vi "Calculate angle of intersection(Circle).vi"(8 "error in (no error)":errorcluster, 9 "Circle":T1, 10 "Pixel density":dbl format="%#_13g", 11 "Input point":cluster{"X":sgl, "Y":sgl}) -> (0 "error out":errorcluster, 1 "Sleeping line start point":cluster{"X":sgl, "Y":sgl}, 2 "slanting line start poing":cluster{"X":sgl, "Y":sgl}, 3 "Angle":sgl)   [LabVIEW 2019]
uses:
  <vilib>/vision/NI_Vision_Development_Module.lvlib
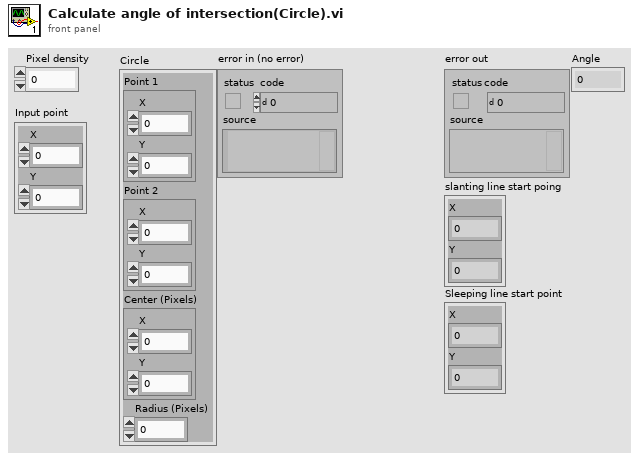
[diagram p1: front panel]
types:
  T1 = cluster{"Point 1":cluster{"X":sgl, "Y":sgl}, "Point 2":cluster{"X":sgl, "Y":sgl}, "Center (Pixels)":cluster{"X":sgl, "Y":sgl}, "Radius (Pixels)":dbl}
  T2 = cluster{"Origin":cluster{"X":sgl, "Y":sgl}, "Angle (deg)":sgl, "Axis Reference":u32}
  T3 = typedef "ROI Descriptor" = cluster{"Global Rectangle":i32[], "Contours":cluster{"ID":enum32{"External", "Internal"}, "Type":u32, "Coordinates":i32[]}[]}
  T4 = typedef "IMAQ Point" = cluster{"X":sgl, "Y":sgl}
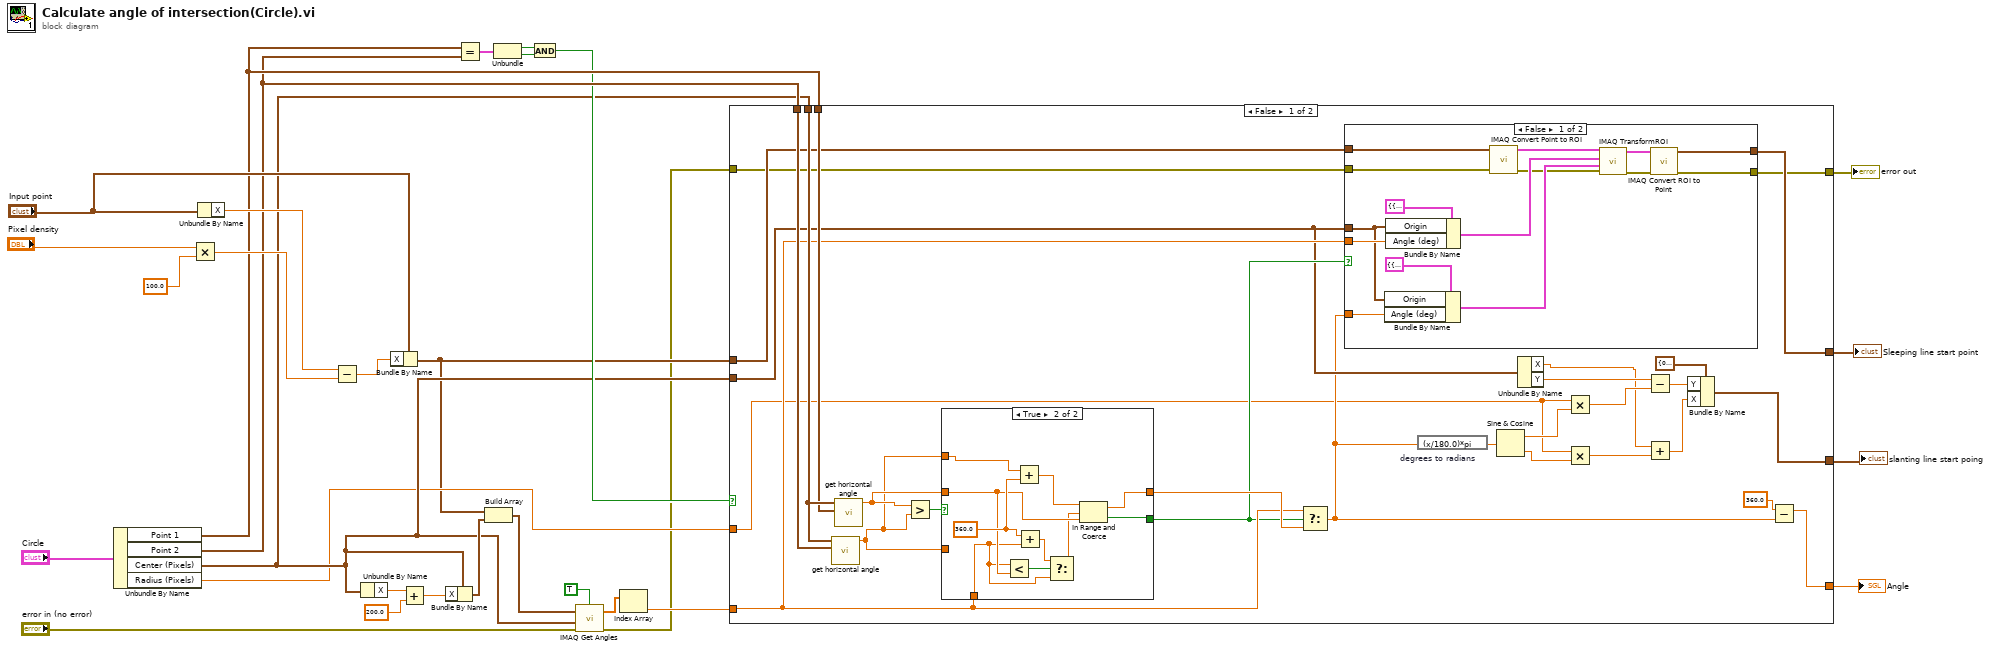
[diagram p0: block diagram]
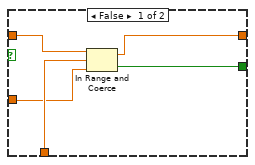
[diagram p3: hidden frame]
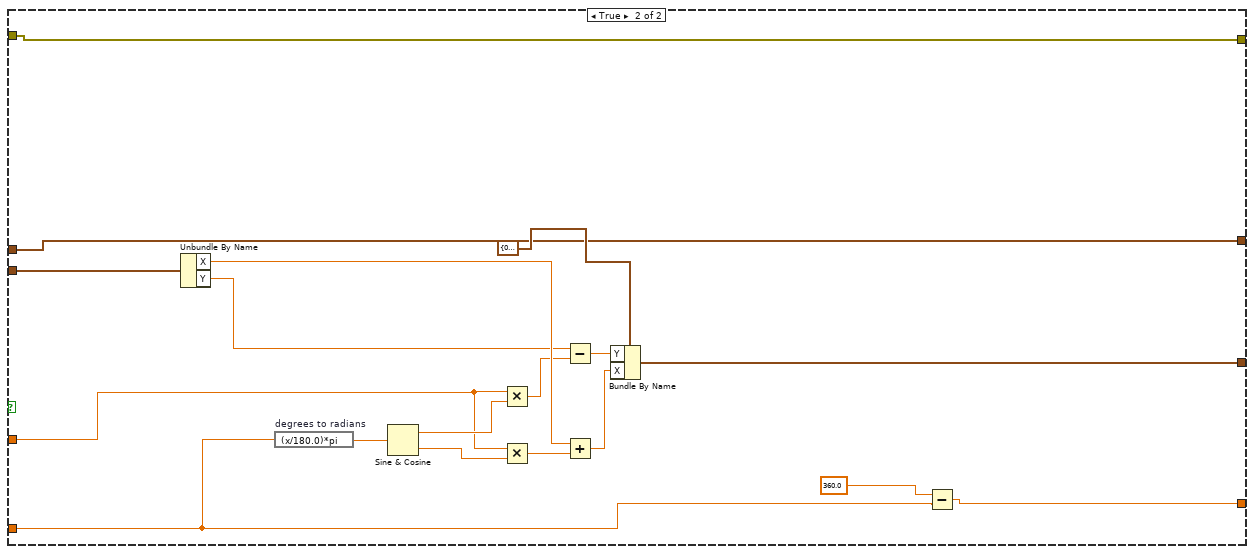
[diagram p4: hidden frame]
diagram:
  n1 = Unbundle By Name("Circle") -> ("Point 1"=w15:cluster{"X":sgl, "Y":sgl}, "Point 2"=w14:cluster{"X":sgl, "Y":sgl}, "Center (Pixels)"=w8:cluster{"X":sgl, "Y":sgl}, "Radius (Pixels)"=w7:dbl)
  n2 = Multiply(x="Pixel density", y=100.0) -> (x*y=w27:dbl)
  n3 = Unbundle By Name("Input point") -> ("X"=w28:sgl)
  n4 = Subtract(x=w28, y=w27) -> (x-y=w25:dbl)
  n5 = Unbundle By Name(w8) -> ("X"=w23:sgl)
  n6 = Bundle By Name(cluster="Input point", "X"=w25) -> (w5:cluster{"X":sgl, "Y":sgl})
  n7 = Add(x=w23, y=sgl 200.0) -> (x+y=w21:sgl)
  n8 = Bundle By Name(cluster=w8, "X"=w21) -> (w19:cluster{"X":sgl, "Y":sgl})
  n9 = Equal?(x=w15, y=w14) -> (x = y?=w13:cluster{"X":bool, "Y":bool})
  n10 = Build Array(w5, w19) -> (w20:cluster{"X":sgl, "Y":sgl}[])
  n11 = Unbundle(w13) -> ("X"=w12:bool, "Y"=w11:bool)
  n12 = And(x=w12, y=w11) -> (x .and. y?=w10:bool)
  n13 = call "IMAQ Get Angles"("error in (no error)"="error in (no error)", "Vertex"=w8, "Points"=w20, "Use Vertex (No)"=TRUE) -> ("error out"=w2:errorcluster, "Angles (deg)"=w16:sgl[])  [unwired: 1 in, 1 out]
  n14 = Index Array(array=w16) -> (element=w6:sgl)  [unwired: 1 in]
  n15 = case shown="False" w10 {
    tunnel: w6 -> [w53 w94]
    tunnel: w8 -> [w57 _]
    tunnel: w15 -> [w56 _]
    tunnel: w14 -> [w55 _]
    tunnel: [w52 w93] -> w9
    tunnel: w8 -> [w34 w99]
    tunnel: w7 -> [w32 w98]
    tunnel: [w35 w97] -> w3
    tunnel: w5 -> [w49 w96]
    tunnel: [w48 w96] -> w4
    tunnel: w2 -> [w47 w95]
    tunnel: [w46 w95] -> w1
    frame False {
      n16 = call "get horizontal angle.vi"("Point 2"=w55, "Point 1"=w57) -> ("Angle w.r.t horizontal\n(in degrees)"=w31:sgl)  [unwired: 9 in]
      n17 = call "get horizontal angle.vi"("Point 2"=w56, "Point 1"=w57) -> ("Angle w.r.t horizontal\n(in degrees)"=w58:sgl)  [unwired: 9 in]
      n18 = Greater?(x=w58, y=w31) -> (0:w59:bool)
      n19 = case shown="True" w59 {
        tunnel: w58 -> [w81 w86]
        tunnel: w53 -> [w80 w84]
        tunnel: w31 -> [_ w89]
        tunnel: w31 -> [w79 _]
        tunnel: [w77 w90] -> w54
        tunnel: [w78 w91] -> w50
        frame False {
          n20 = In Range and Coerce(upper limit=w81, x=w80, lower limit=w79) -> (coerced(x)=w77:sgl, In Range?=w78:bool)
        }
        frame True {
          w87 = sgl 360.0 ("y")
          n21 = Less?(x=w84, y=w86) -> (x < y?=w85:bool)
          n22 = Add(x=w89, y=w87) -> (x+y=w88:sgl)
          n23 = Add(x=w87, y=w84) -> (x+y=w83:sgl)
          n24 = Select(t=w83, s=w85, f=w84) -> (s? t:f=w82:sgl)
          n25 = In Range and Coerce(upper limit=w88, x=w82, lower limit=w86) -> (coerced(x)=w90:sgl, In Range?=w91:bool)
        }
      }
      n26 = Select(t=w53, s=w50, f=w54) -> (s? t:f=w33:sgl)
      n27 = case shown="False" w50 {
        tunnel: w34 -> [w64 _]
        tunnel: w53 -> [w72 _]
        tunnel: w33 -> [w65 _]
        tunnel: w49 -> [w71 w76]
        tunnel: [w63 w76] -> w48
        tunnel: w47 -> [w62 w75]
        tunnel: [w60 w75] -> w46
        frame False {
          n28 = Bundle By Name(cluster=T2 {"Origin"={"X"=0.0, "Y"=0.0}, "Angle (deg)"=0.0, "Axis Reference"=0} ("Base Reference"), "Origin"=w64, "Angle (deg)"=w65) -> (w68:T2)
          n29 = Bundle By Name(cluster=T2 {"Origin"={"X"=0.0, "Y"=0.0}, "Angle (deg)"=0.0, "Axis Reference"=0} ("Base Reference"), "Origin"=w64, "Angle (deg)"=w72) -> (w69:T2)
          n30 = call "IMAQ Convert Point to ROI"("error in (no error)"=w62, "Point"=w71) -> ("error out"=w61:errorcluster, "ROI Descriptor"=w70:T3)  [unwired: 7 in]
          n31 = call "IMAQ TransformROI"("error in (no error)"=w61, "New Reference"=w68, "Base Reference"=w69, "ROI Descriptor"=w70) -> ("error out"=w67:errorcluster, "ROI Descriptor out"=w66:T3)  [unwired: 6 in]
          n32 = call "IMAQ Convert ROI to Point"("error in (no error)"=w67, "ROI Descriptor"=w66) -> ("error out"=w60:errorcluster, "Point"=w63:T4)  [unwired: 7 in]
        }
        frame True {
        }
      }
      n33 = expression code="(x/180.0)*pi" "degrees to radians"(w33) -> (w45:sgl)
      n34 = Sine & Cosine(0:w45) -> (1:w44:sgl, 2:w43:sgl)
      n35 = Unbundle By Name(w34) -> ("X"=w37:sgl, "Y"=w41:sgl)
      n36 = Multiply(x=w32, y=w44) -> (x*y=w42:dbl)
      n37 = Multiply(x=w32, y=w43) -> (x*y=w40:dbl)
      n38 = Subtract(x=w41, y=w42) -> (x-y=w39:dbl)
      n39 = Add(x=w37, y=w40) -> (x+y=w38:dbl)
      n40 = Bundle By Name(cluster=cluster{"X":sgl, "Y":sgl} {"X"=0.0, "Y"=0.0} ("output cluster"), "Y"=w39, "X"=w38) -> (w35:cluster{"X":sgl, "Y":sgl})
      n41 = Subtract(x=sgl 360.0, y=w33) -> (x-y=w52:sgl)
    }
    frame True {
      n42 = Unbundle By Name(w99) -> ("X"=w105:sgl, "Y"=w104:sgl)
      n43 = expression code="(x/180.0)*pi" "degrees to radians"(w94) -> (w100:sgl)
      n44 = Sine & Cosine(0:w100) -> (1:w101:sgl, 2:w102:sgl)
      n45 = Multiply(x=w98, y=w101) -> (x*y=w103:dbl)
      n46 = Multiply(x=w98, y=w102) -> (x*y=w106:dbl)
      n47 = Subtract(x=w104, y=w103) -> (x-y=w108:dbl)
      n48 = Add(x=w105, y=w106) -> (x+y=w109:dbl)
      n49 = Bundle By Name(cluster=cluster{"X":sgl, "Y":sgl} {"X"=0.0, "Y"=0.0} ("output cluster"), "Y"=w108, "X"=w109) -> (w97:cluster{"X":sgl, "Y":sgl})
      n50 = Subtract(x=sgl 360.0, y=w94) -> (x-y=w93:sgl)
    }
  }
  "error out" <- w1
  "Angle" <- w9
  "Sleeping line start point" <- w4
  "slanting line start poing" <- w3
